vi "Destroy User Events.vi"(11 "Panel in":refnum<class "Panel.lvclass">) -> (0 "error out":errorcluster)   [LabVIEW 2021, in "Panel.lvclass"]
uses:
  Panel.lvclass
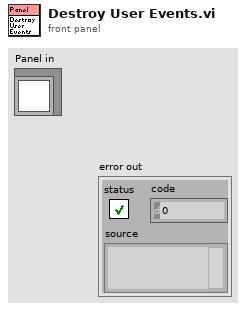
[diagram p1: front panel]
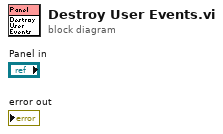
[diagram p0: block diagram]
diagram:
